vi "Template Dut TxRx Configure.vi"(0 "Dut Handle in":T2, 5 "niDTS GNSS DUT Parameters":T1, 11 "error in (no error)":errorcluster) -> (4 "Dut Handle out":T2, 15 "error out":errorcluster)   [LabVIEW 2014, in "niDTS Template.lvlib"]
doc: "Set the basic parameters for the WLAN TX Test. \n\nInputs:\n* Apply Additional Defaults. This allows more advanced parameters, which are dependant on the inputs, to have their default values set.\n\nCallbacks:\n* WLAN DUT Additional Defaults\n\nNote: This behavior is expected to be depricated when full parameter sets are passed as inputs and the input dependant defaults are calculated on the top parameter setting level."
uses:
  niDTS Template.lvlib
  Framework/Dut/Includes/niDTS Dut INC Handle.ctl
  Framework/Dut/Objects/BASE_class/niDTS Dut.lvclass
  Includes/Template Dut INC Parameters.ctl
  Includes/Template Dut INC Handle.ctl
  Objects/BASE_class/Template Dut.lvclass
  Framework/Logger/Objects/BASE_class/niDTS Logger.lvclass
  Framework/niDTS Framework.lvlib
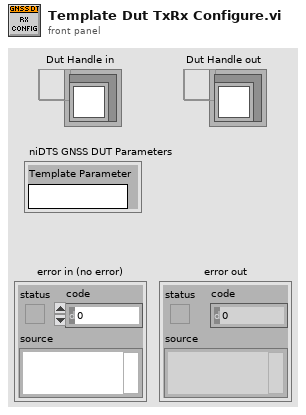
[diagram p1: front panel]
types:
  T1 = typedef "niDTS Template.lvlib/Template Dut INC Parameters.ctl" = cluster{"Template Parameter":string}
  T2 = typedef "niDTS Framework.lvlib/niDTS Dut INC Handle.ctl" = refnum<data-value>
  T3 = typedef "niDTS Template.lvlib/Template Dut INC Handle.ctl" = refnum<data-value>
  T4 = typedef "niDTS Framework.lvlib/niDTS Logger INC Handle.ctl" = refnum<data-value>
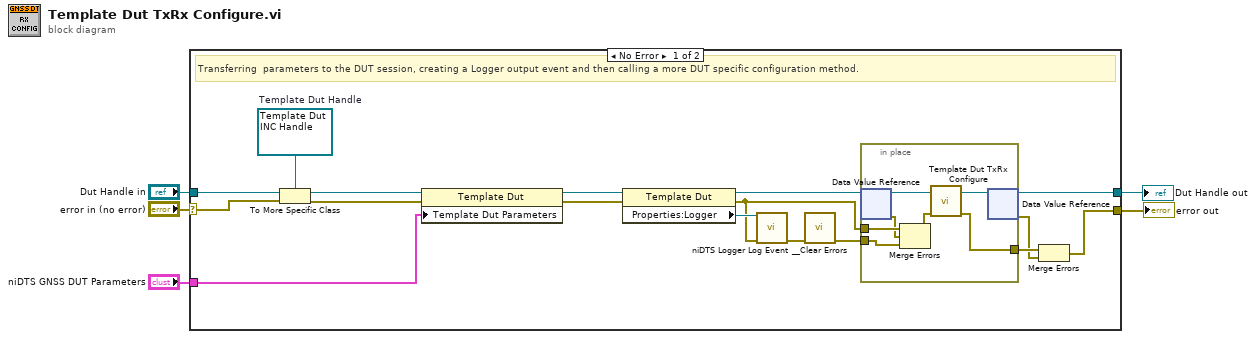
[diagram p0: block diagram]
diagram:
  n1 = case shown="No Error" "error in (no error)" {
    selector: "error in (no error)" -> [w21 w30]
    tunnel: "Dut Handle in" -> [w22 w31]
    tunnel: [w20 w31] -> w4
    tunnel: [w19 w30] -> w3
    tunnel: "niDTS GNSS DUT Parameters" -> [w11 _]
    frame No Error {
      w16 = T3 refnum  # Template Dut Handle
      # "Transferring  parameters to the DUT session, creating a Logger output event and then calling a more DUT specific configuration method."
      n2 = To More Specific Class(target class=w16, reference=w22, error in=w21) -> (specific class reference=w15:T3, error out=w13:errorcluster)
      n3 = property class="Template Dut"(reference=w15, error in=w13, "Template Dut Parameters"=w11) -> (reference out=w14:T3, error out=w12:errorcluster)
      n4 = property class="Template Dut"(reference=w14, error in=w12) -> (reference out=w17:T3, error out=w8:errorcluster, "Properties:Logger"=w18:T4)
      n5 = call "niDTS Logger Log Event.vi"("Logger Handle"=w18, "error in (no error)"=w8) -> ("error out"=w7:errorcluster)  [unwired: 11 in, 2 out]
      n6 = call "__Clear Errors.vi"("error in (no error)"=w7) -> ("error out"=w6:errorcluster)  [unwired: 5 in, 1 out]
      n7 = in-place {
        in-place-border: w8 -> [w25]
        in-place-border: [w26] -> w10
        in-place-border: w6 -> [w23]
        n8 = in-place-dvr #1(w17) -> (w29:refnum<class "Template Dut.lvclass">, w24:errorcluster)
        n9 = Merge Errors(w25, w24, w23) -> (w28:errorcluster)
        n10 = call-dynamic "Template Dut TxRx Configure.vi"("Template Dut in"=w29, "error in (no error)"=w28) -> ("Template Dut out"=w27:refnum<class "Template Dut.lvclass">, "error out"=w26:errorcluster)  [unwired: 12 in]
        n11 = in-place-dvr #1(w27) -> (w20:T3, w9:errorcluster)
      }
      n12 = Merge Errors(w10, w9) -> (w19:errorcluster)
    }
    frame Error {
    }
  }
  "error out" <- w3
  "Dut Handle out" <- w4
